vi "AngularVelocityChecker.vi"() -> ()   [LabVIEW 2014]
uses:
  <vilib>/NXT/Block Support/NXT_OutputPort.ctl
  <vilib>/NXT/NXTIO Xnodes/NXTIONodeSubVIs/LEGOMotorStatus.vi
  <vilib>/NXT/NXTIO Xnodes/NXTIONodeSubVIs/NXTCheckBattery.vi
  <vilib>/NXT/NXTIO Xnodes/NXTIONodeSubVIs/NXTMoveMotors.vi
  <vilib>/NXT/NXTIO Xnodes/AddressXNode/NXTIOAddress.xnode
  <vilib>/NXT/Subs/LVHSConnector.ctl
  <vilib>/NXT/NXTIO Xnodes/NXTIOXNode/NXTIO.xnode
  <vilib>/NXT/LegoClasses/BrickReference/BrickReference.lvclass
panel:
  out "Voltage":sgl
  out "deg/s":dbl
  out "rad/s":dbl
  in  "모터 값":i8
  in  "모터 번호":i32
  out "시간 (ms)":i32
  out "엔코더 값":i32
  # "모터 번호 1 : w1\n모터 번호 2 : w2"
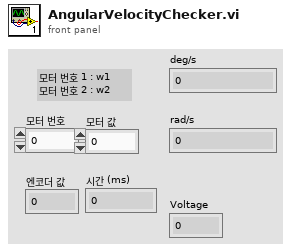
[diagram p1: front panel]
types:
  T1 = typedef "NXT_OutputPort.ctl" = u8
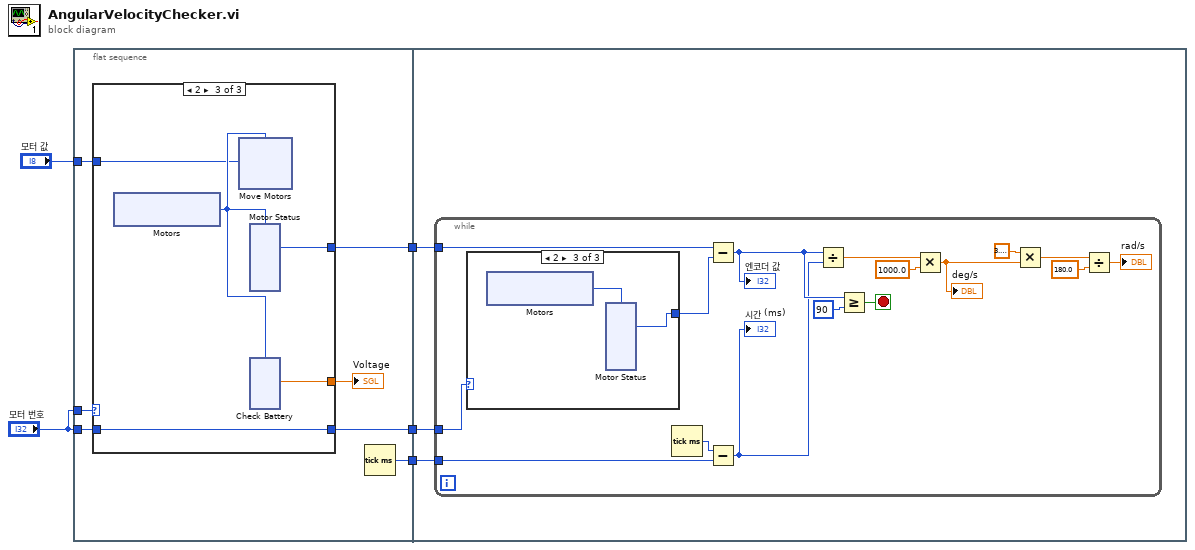
[diagram p0: block diagram]
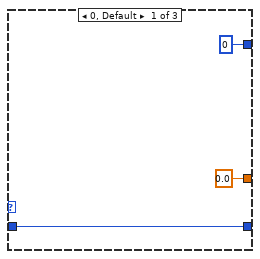
[diagram p2: hidden frame]
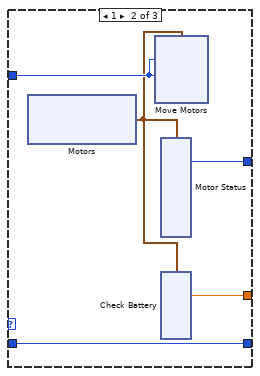
[diagram p3: hidden frame]
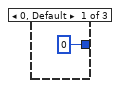
[diagram p4: hidden frame]
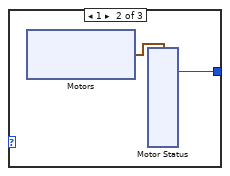
[diagram p5: hidden frame]
diagram:
  n1 = flat-sequence {
    tunnel: "모터 번호" -> [w12]
    tunnel: "모터 값" -> [w11]
    tunnel: [w10] -> w4
    tunnel: [w9] -> w3
    tunnel: "모터 번호" -> [w8]
    tunnel: [w7] -> w1
    tunnel: w4 -> [w73]
    tunnel: w3 -> [w72]
    tunnel: w1 -> [w71]
    frame #0 {
      n2 = case shown="2" w12 {
        tunnel: w11 -> [_ w20 w45]
        tunnel: [w15 w19 w49] -> w9
        tunnel: w8 -> [w15 w19 w49]
        tunnel: [0 ("Position 1") w18 w47] -> w7
        tunnel: [sgl 0.0 ("Voltage 1") w16 w46] -> w6
        frame 0, Default {
        }
        frame 1 {
          n3 = xnode "Motors"() -> ("Motor"=w17:cluster{"Port":T1, "Port":T1})
          n4 = xnode "Move Motors"("Power/Speed 2"=w20, "Power/Speed 1"=w20, "Motors"=w17) -> ()  [unwired: 1 in, 1 out]
          n5 = xnode "Motor Status"("Motors"=w17) -> ("Position 1"=w18:i32)  [unwired: 1 in, 4 out]
          n6 = xnode "Check Battery"("Motors"=w17) -> ("Voltage 1"=w16:sgl)  [unwired: 1 in, 2 out]
        }
        frame 2 {
          n7 = xnode "Motors"() -> ("Motor"=w48:T1)
          n8 = xnode "Move Motors"("Power/Speed 1"=w45, "Motors"=w48) -> ()  [unwired: 1 in, 1 out]
          n9 = xnode "Motor Status"("Motors"=w48) -> ("Position 1"=w47:i32)  [unwired: 1 in, 2 out]
          n10 = xnode "Check Battery"("Motors"=w48) -> ("Voltage 1"=w46:sgl)  [unwired: 1 in, 1 out]
        }
      }
      "Voltage" <- w6
      n11 = Tick Count (ms)() -> (millisecond timer value=w10:u32)
    }
    frame #1 {
      n12 = while {
        tunnel: w73 -> [w88]
        tunnel: w72 -> [w87]
        tunnel: w71 -> [w85]
        stop <- w83 stop-if-true
        n13 = case shown="2" w87 {
          tunnel: [0 ("Position 1") w91 w105] -> w86
          frame 0, Default {
          }
          frame 1 {
            n14 = xnode "Motors"() -> ("Motor"=w92:cluster{"Port":T1, "Port":T1})
            n15 = xnode "Motor Status"("Motors"=w92) -> ("Position 1"=w91:i32)  [unwired: 1 in, 4 out]
          }
          frame 2 {
            n16 = xnode "Motors"() -> ("Motor"=w104:T1)
            n17 = xnode "Motor Status"("Motors"=w104) -> ("Position 1"=w105:i32)  [unwired: 1 in, 2 out]
          }
        }
        n18 = Tick Count (ms)() -> (millisecond timer value=w89:u32)
        n19 = Subtract(x=w85, y=w86) -> (x-y=w82:i32)
        "엔코더 값" <- w82
        n20 = Subtract(x=w89, y=w88) -> (x-y=w81:u32)
        "시간 (ms)" <- w81
        n21 = Divide(x=w82, y=w81) -> (x/y=w80:dbl)
        n22 = Greater Or Equal?(x=w82, y=90) -> (x >= y?=w83:bool)
        n23 = Multiply(x=w80, y=1000.0) -> (x*y=w78:dbl)
        "deg/s" <- w78
        n24 = Multiply(x=3.141592653589793, y=w78) -> (x*y=w75:dbl)
        n25 = Divide(x=w75, y=180.0) -> (x/y=→"rad/s":dbl)
      }
    }
  }
